vi "用户登录.vi"() -> (0 "管理人员1+密码":string[][](array[string]), 1 "管理人员-T存在-F不存在":bool, 2 "操作人员0+密码":string[][](array[string]), 3 "操作人员-T存在-F不存在":bool, 4 "T正常-F错误":bool, 5 "用户类别_out":u8, 6 "用户名的顺序out":u16, 7 "密码文件路径":path)   [LabVIEW 2018]
doc: "密码输入对话框"
panel:
  in  "用户名":u16(ring) items=["a", "b", "c"]
  in  "用户类别":u8(ring) items=["操作人员", "管理人员"]
  in  "退出":bool
  in  "登录":bool
  in  "请输入密码":string
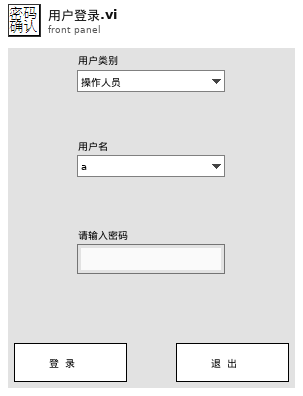
[diagram p1: front panel]
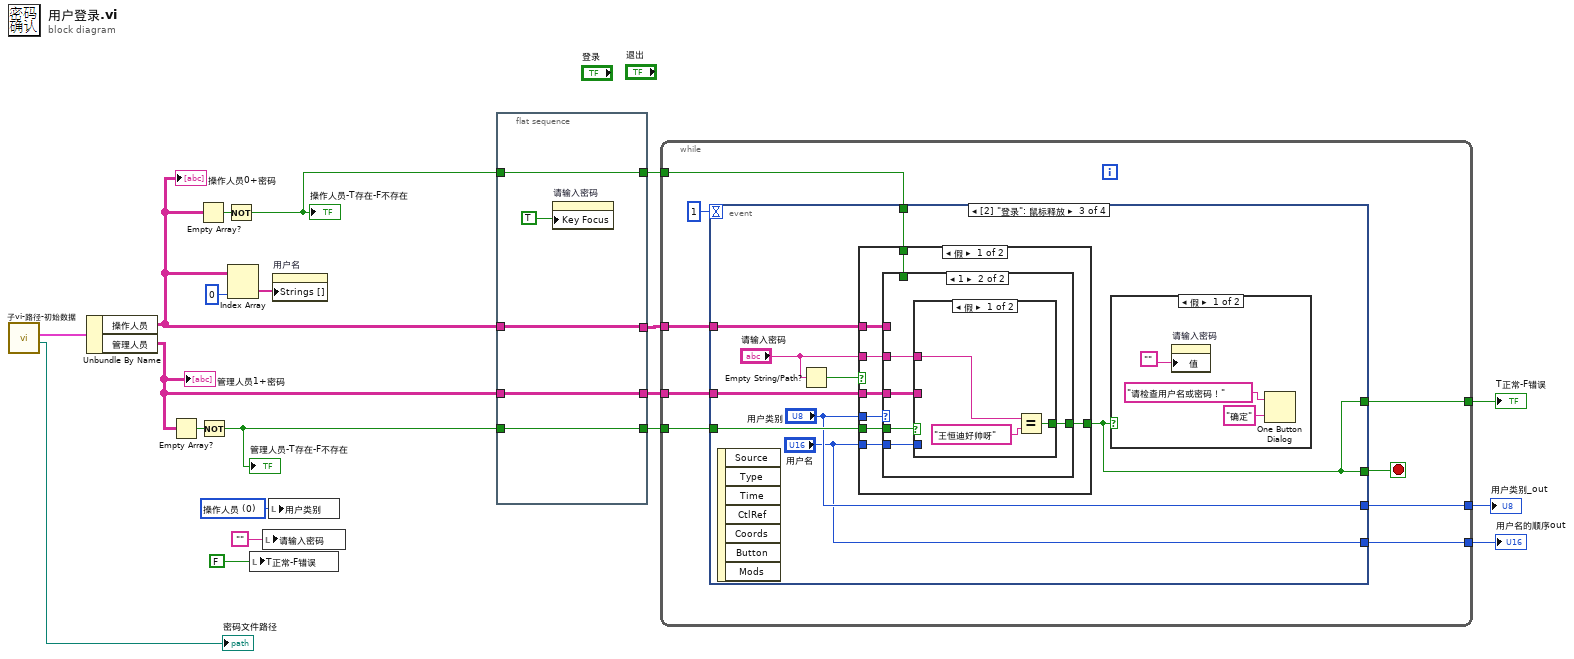
[diagram p0: block diagram]
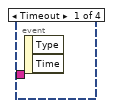
[diagram p2: hidden frame]
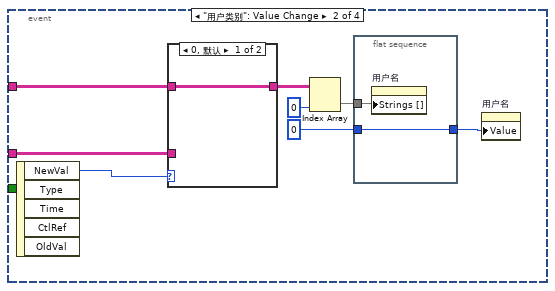
[diagram p3: hidden frame]
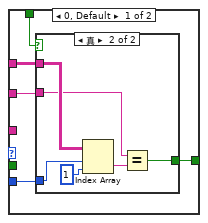
[diagram p5: hidden frame]
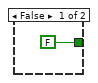
[diagram p6: hidden frame]
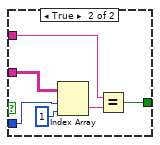
[diagram p7: hidden frame]
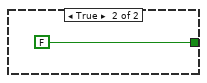
[diagram p8: hidden frame]
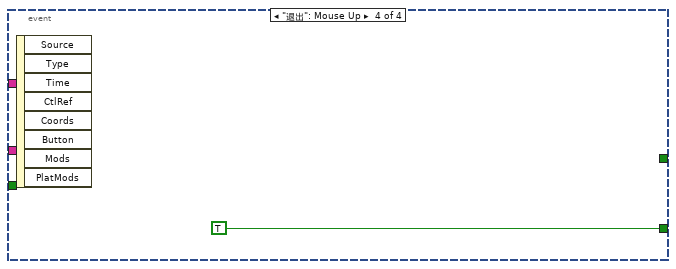
[diagram p10: hidden frame]
diagram:
  w17 = u8 0 items=["操作人员", "管理人员"] ("人员类别")
  n1 = call "子vi-路径-初始数据.vi"() -> ("密码文件路径"=→"密码文件路径":path, "用户名密码"=w16:cluster{"操作人员":string[][], "管理人员":string[][]})  [unwired: 8 in, 2 out]
  n2 = Unbundle By Name(w16) -> ("操作人员"=w8:string[][], "管理人员"=w6:string[][])
  "操作人员0+密码" <- w8
  "管理人员1+密码" <- w6
  n3 = Empty Array?(array=w6) -> (empty?=w13:bool)
  n4 = Empty Array?(array=w8) -> (empty?=w15:bool)
  n5 = Not(x=w13) -> (.not. x?=w4:bool)
  "管理人员-T存在-F不存在" <- w4
  n6 = Not(x=w15) -> (.not. x?=w10:bool)
  "操作人员-T存在-F不存在" <- w10
  n7 = Index Array(array=w8, index (col)=0 ("禁用的索引 (col)")) -> (element=w20:string[])  [unwired: 1 in]
  n8 = local write "T正常-F错误"(FALSE ("T退出-F正常进行")) -> ()
  n9 = local write "请输入密码"("") -> ()
  n10 = local write "用户类别"(w17) -> ()
  n11 = property on="用户名" class="Ring (严格)"("Strings []"=w20) -> ()  [unwired: 2 in, 2 out]
  n12 = flat-sequence {
    tunnel: [w24] -> w9
    tunnel: w10 -> [w24]
    tunnel: [w23] -> w7
    tunnel: w8 -> [w23]
    tunnel: [w22] -> w5
    tunnel: w6 -> [w22]
    tunnel: [w21] -> w3
    tunnel: w4 -> [w21]
    frame #0 {
      n13 = property on="请输入密码" class="Str"("Key Focus"=TRUE ("键选中")) -> ()  [unwired: 2 in, 2 out]
    }
  }
  n14 = while {
    tunnel: w7 -> [w33]
    tunnel: w5 -> [w32]
    tunnel: w3 -> [w31]
    tunnel: w9 -> [w30]
    tunnel: [w29] -> w12
    tunnel: [w28] -> w11
    tunnel: [w27] -> w2
    stop <- w34 stop-if-true
    n15 = event shown="[2] \"登录\": 鼠标释放" {
      selector: _ -> [_ _ _ _]
      dyn-events: _ -> [_ _ _ _]
      timeout: 1 -> [_ _ _ _]
      tunnel: [_ _ w47 TRUE] -> w34
      tunnel: w33 -> [_ w42 w55 _]
      tunnel: w32 -> [_ w39 w54 _]
      tunnel: [_ _ "用户类别" _] -> w29
      tunnel: w31 -> [_ _ w53 _]
      tunnel: w30 -> [_ _ w52 _]
      tunnel: [_ _ "用户名" _] -> w28
      tunnel: [_ _ w47 _] -> w27
      event Timeout {
        n16 = event-data() -> ()  [unwired: 1 in, 2 out]
      }
      event "用户类别": Value Change {
        n17 = event-data() -> ("NewVal"=w38:u8)  [unwired: 1 in, 4 out]
        n18 = case shown="0, 默认" w38 {
          tunnel: w42 -> [w45 _]
          tunnel: [w45 w46] -> w40
          tunnel: w39 -> [_ w46]
          frame 0, Default {
          }
          frame 1 {
          }
        }
        n19 = Index Array(array=w40, index (col)=0 ("禁用的索引 (col)")) -> (element=w41:string[])  [unwired: 1 in]
        n20 = flat-sequence {
          tunnel: w41 -> [w44]
          tunnel: [w43] -> w35
          tunnel: u16 0 ("禁用的索引 (col)") -> [w43]
          frame #0 {
            n21 = property on="用户名" class="Ring (严格)"("Strings []"=w44) -> ()  [unwired: 2 in, 2 out]
          }
        }
        n22 = property on="用户名" class="Ring (严格)"("Value"=w35) -> ()  [unwired: 2 in, 2 out]
      }
      event "登录": Mouse Up {
        n23 = event-data() -> ()  [unwired: 1 in, 7 out]
        n24 = Empty String/Path?(string/path="请输入密码") -> (empty?=w48:bool)
        n25 = case shown="假" w48 {
          tunnel: w55 -> [w63 _]
          tunnel: w54 -> [w62 _]
          tunnel: [w61 FALSE] -> w47
          tunnel: w53 -> [w60 _]
          tunnel: w52 -> [w59 _]
          tunnel: "用户类别" -> [w58 _]
          tunnel: "用户名" -> [w57 _]
          tunnel: "请输入密码" -> [w56 _]
          frame False {
            n26 = case shown="1" w58 {
              tunnel: w63 -> [w67 _]
              tunnel: w62 -> [_ w79]
              tunnel: w56 -> [w68 w78]
              tunnel: w57 -> [w66 w77]
              tunnel: [w64 w76] -> w61
              tunnel: w60 -> [_ w80]
              tunnel: w59 -> [w65 _]
              frame 0, Default {
                n27 = case shown="真" w65 {
                  tunnel: w67 -> [_ w73]
                  tunnel: w68 -> [_ w72]
                  tunnel: w66 -> [_ w71]
                  tunnel: [FALSE w70] -> w64
                  frame False {
                  }
                  frame True {
                    n28 = Index Array(array=w73, index (row)=w71, index (col)=1 ("禁用的索引 (col)")) -> (element=w75:string)
                    n29 = Equal?(x=w72, y=w75) -> (x = y?=w70:bool)
                  }
                }
              }
              frame 1 {
                n30 = case shown="假" w80 {
                  tunnel: w79 -> [_ w87]
                  tunnel: w78 -> [w83 w86]
                  tunnel: w77 -> [_ w85]
                  tunnel: [w81 w84] -> w76
                  frame False {
                    n31 = Equal?(x=w83, y="王恒迪好帅呀") -> (x = y?=w81:bool)
                  }
                  frame True {
                    n32 = Index Array(array=w87, index (row)=w85, index (col)=1 ("禁用的索引 (col)")) -> (element=w89:string)
                    n33 = Equal?(x=w86, y=w89) -> (x = y?=w84:bool)
                  }
                }
              }
            }
          }
          frame True {
          }
        }
        n34 = case shown="假" w47 {
          frame False {
            n35 = property on="请输入密码" class="Str"("值"="") -> ()  [unwired: 2 in, 2 out]
            n36 = One Button Dialog(message="请检查用户名或密码！", button name ("OK")="确定") -> ()  [unwired: 1 out]
          }
          frame True {
          }
        }
      }
      event "退出": Mouse Up {
        n37 = event-data() -> ()  [unwired: 1 in, 8 out]
      }
    }
  }
  "用户类别_out" <- w12
  "用户名的顺序out" <- w11
  "T正常-F错误" <- w2
